vi "SetSmoothingMode.vi"(8 "error in (no error)":errorcluster, 10 "SmoothingMode":T1, 11 "CreateGraphics in":refnum<k24>) -> (0 "error out":errorcluster, 3 "CreateGraphics out":refnum<k24>)   [LabVIEW 2020, in "LcPictureBox.lvclass"]
uses:
  LcPictureBox.lvclass
  System.Drawing
  SmoothingMode.ctl
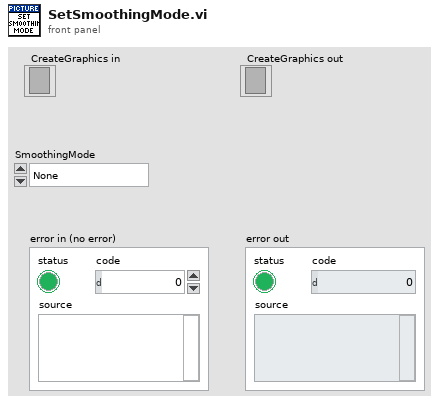
[diagram p1: front panel]
types:
  T1 = typedef "LcPictureBox.lvclass/SmoothingMode.ctl" = enum16{"None", "HighSpeed", "HighQuality", "AntiAlias"}
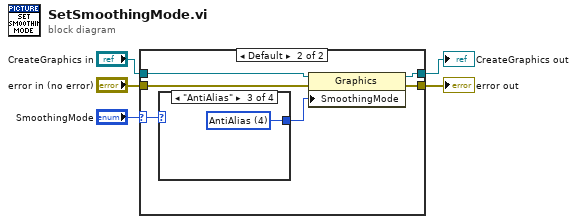
[diagram p0: block diagram]
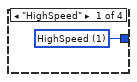
[diagram p3: hidden frame]
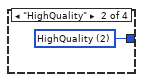
[diagram p4: hidden frame]
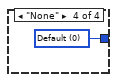
[diagram p5: hidden frame]
diagram:
  n1 = case shown="Default" "SmoothingMode" {
    selector: "SmoothingMode" -> [_ w8]
    tunnel: "CreateGraphics in" -> [w6 w13]
    tunnel: "error in (no error)" -> [w7 w12]
    tunnel: [w7 w11] -> w3
    tunnel: [w6 w10] -> w4
    frame "None" {
    }
    frame Default {
      n2 = case shown="\"AntiAlias\"" w8 {
        tunnel: [w14 w15 w16 w17] -> w9
        frame "HighSpeed" {
          w14 = 1 items=["Default"=0, "HighSpeed"=1, "HighQuality"=2, "None"=3, "AntiAlias"=4, "Invalid"=-1] ("SmoothingMode")
        }
        frame "HighQuality" {
          w15 = 2 items=["Default"=0, "HighSpeed"=1, "HighQuality"=2, "None"=3, "AntiAlias"=4, "Invalid"=-1] ("SmoothingMode")
        }
        frame "AntiAlias" {
          w16 = 4 items=["Default"=0, "HighSpeed"=1, "HighQuality"=2, "None"=3, "AntiAlias"=4, "Invalid"=-1] ("SmoothingMode")
        }
        frame "None" {
          w17 = 0 items=["Default"=0, "HighSpeed"=1, "HighQuality"=2, "None"=3, "AntiAlias"=4, "Invalid"=-1] ("SmoothingMode")
        }
      }
      n3 = property class="Graphics"(reference=w13, error in=w12, "SmoothingMode"=w9) -> (reference out=w10:refnum<k24>, error out=w11:errorcluster)
    }
  }
  "CreateGraphics out" <- w4
  "error out" <- w3
